vi "ep_Update Config Info (Waveform).vi"(6 "data length":i32, 7 "timing info":cluster{"t0":timestamp, "fs":sgl}, 8 "error in":errorcluster, 11 "task in":T1={"file refnums"=[], "Data Object"=refnum, "config info"={"station_name"="", "rec_dev_id"="", "rev_year"=1999.0, "TT"=0, "##A"=0, "##D"=0, "analog channel info"=[], "status channel info"=[], "lf"=-inf, "nrates"=65535, "samp info"=[], "initial timestamp"=timestamp(0 s since 1904-01-01), "trigger timestamp"=timestamp(0 s since 1904-01-01), "ft"=enum."Binary", "timemult"=1.0}, "public inf content"={"Source"="", "Record Type"=enum."Fault", "Phase ID"="", "Event Description"="", "Device ID"="", "Distance of Fault"=-1.0, "Distance Unit"=enum."Miles", "Max_Current"=inf, "Min_Current"=-inf, "Max_Voltage"=inf, "Min_Voltage"=-inf, "EventNoteCount"=0, "Event Information"=[]}, "private inf content"=[], "internal buffers"={"start index"=1, "config to public inf"=enum."disabled", "static config info"="", "static file_des record inf"="", "static file_des channel inf"="", "public inf"="", "private inf"=""}} {"public inf content"."Event Information"."min sample number" max=9999999999; "public inf content"."Event Information"."max sample number" max=9999999999; "config info"."nrates" max=999; "config info"."status channel info"."Dn" min=1 max=999999; "config info"."analog channel info"."An" min=1 max=999999; "config info"."trigger timestamp" format="%<%H:%M:%S%6u\n%d/%m/%Y>T"; "config info"."initial timestamp" format="%<%H:%M:%S%6u\n%d/%m/%Y>T"; "config info"."##D" max=999999; "config info"."##A" max=999999; "config info"."TT" min=1 max=999999; "config info"."rev_year" min=1999.0 max=1999.0}) -> (0 "error out":errorcluster, 3 "task out":T1={"file refnums"=[], "Data Object"=refnum, "config info"={"station_name"="", "rec_dev_id"="", "rev_year"=1999.0, "TT"=0, "##A"=0, "##D"=0, "analog channel info"=[], "status channel info"=[], "lf"=-inf, "nrates"=65535, "samp info"=[], "initial timestamp"=timestamp(0 s since 1904-01-01), "trigger timestamp"=timestamp(0 s since 1904-01-01), "ft"=enum."Binary", "timemult"=1.0}, "public inf content"={"Source"="", "Record Type"=enum."Fault", "Phase ID"="", "Event Description"="", "Device ID"="", "Distance of Fault"=-1.0, "Distance Unit"=enum."Miles", "Max_Current"=inf, "Min_Current"=-inf, "Max_Voltage"=inf, "Min_Voltage"=-inf, "EventNoteCount"=0, "Event Information"=[]}, "private inf content"=[], "internal buffers"={"start index"=1, "config to public inf"=enum."disabled", "static config info"="", "static file_des record inf"="", "static file_des channel inf"="", "public inf"="", "private inf"=""}} {"public inf content"."Event Information"."min sample number" max=9999999999; "public inf content"."Event Information"."max sample number" max=9999999999; "config info"."nrates" max=999; "config info"."status channel info"."Dn" min=1 max=999999; "config info"."analog channel info"."An" min=1 max=999999; "config info"."trigger timestamp" format="%<%H:%M:%S%6u\n%d/%m/%Y>T"; "config info"."initial timestamp" format="%<%H:%M:%S%6u\n%d/%m/%Y>T"; "config info"."##D" max=999999; "config info"."##A" max=999999; "config info"."TT" min=1 max=999999; "config info"."rev_year" min=1999.0 max=1999.0})   [LabVIEW 2011, in "NI_EP_COMTRADE.lvlib"]
uses:
  <vilib>/addons/Electrical Power/File IO/NI_EP_COMTRADE.lvlib
  <vilib>/addons/Electrical Power/File IO/COMTRADE/typedefs/ep_Task.ctl
  <vilib>/addons/Electrical Power/File IO/COMTRADE/typedefs/ep_Config Info.ctl
  <vilib>/addons/Electrical Power/File IO/COMTRADE/typedefs/ep_Analog Channel Info.ctl
  <vilib>/addons/Electrical Power/File IO/COMTRADE/typedefs/ep_Status Channel Info.ctl
  <vilib>/addons/Electrical Power/File IO/COMTRADE/typedefs/ep_File Format.ctl
  <vilib>/addons/Electrical Power/File IO/COMTRADE/typedefs/ep_Public Inf Content.ctl
  <vilib>/addons/Electrical Power/File IO/COMTRADE/typedefs/ep_Public Event Inf.ctl
  <vilib>/addons/Electrical Power/File IO/COMTRADE/typedefs/ep_Private Inf Content.ctl
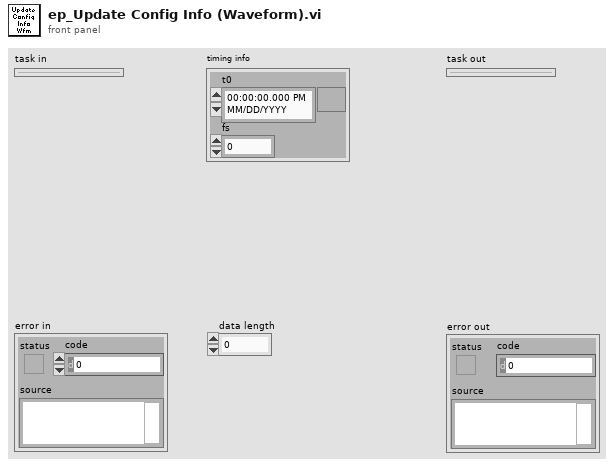
[diagram p1: front panel]
types:
  T1 = typedef "NI_EP_COMTRADE.lvlib/ep_Task.ctl" = cluster{"file refnums":refnum<file>[], "Data Object":refnum<k20>, "config info":T2, "public inf content":T6, "private inf content":T8, "internal buffers":cluster{"start index":u32, "config to public inf":enum16{"disabled", "enabled", "buffered"}, "static config info":string, "static file_des record inf":string, "static file_des channel inf":string, "public inf":string, "private inf":string}}
  T2 = typedef "NI_EP_COMTRADE.lvlib/ep_Config Info.ctl" = cluster{"station_name":string, "rec_dev_id":string, "rev_year":dbl, "TT":u32, "##A":u32, "##D":u32, "analog channel info":T3[], "status channel info":T4[], "lf":sgl, "nrates":u16, "samp info":cluster{"samp":sgl, "endsamp":u32}[], "initial timestamp":timestamp, "trigger timestamp":timestamp, "ft":T5, "timemult":sgl}
  T3 = typedef "NI_EP_COMTRADE.lvlib/ep_Analog Channel Info.ctl" = cluster{"An":u32, "ch_id":string, "ph":string, "ccbm":string, "uu":string, "a":sgl, "b":sgl, "skew":sgl, "min":i32, "max":i32, "primary":sgl, "secondary":sgl, "PS":enum16{"P", "S"}}
  T4 = typedef "NI_EP_COMTRADE.lvlib/ep_Status Channel Info.ctl" = cluster{"Dn":u32, "ch_id":string, "ph":string, "ccbm":string, "Y":bool}
  T5 = typedef "NI_EP_COMTRADE.lvlib/ep_File Format.ctl" = enum16{"ASCII", "Binary"}
  T6 = typedef "NI_EP_COMTRADE.lvlib/ep_Public Inf Content.ctl" = cluster{"Source":string, "Record Type":enum16{"Fault", "Unknown", "Misoperation", "Close", "Trip", "Reclose", "Power swing", "Simulation"}, "Phase ID":string, "Event Description":string, "Device ID":string, "Distance of Fault":dbl, "Distance Unit":enum16{"Miles", "Kilometers", "Percent of line", "Percent of setting", "Ohms"}, "Max_Current":dbl, "Min_Current":dbl, "Max_Voltage":dbl, "Min_Voltage":dbl, "EventNoteCount":u32, "Event Information":T7[]}
  T7 = typedef "NI_EP_COMTRADE.lvlib/ep_Public Event Inf.ctl" = cluster{"channel number":u32, "max value":dbl, "min value":dbl, "max sample number":u64, "min sample number":u64, "max sample text":string[], "min sample text":string[]}
  T8 = typedef "NI_EP_COMTRADE.lvlib/ep_Private Inf Content.ctl" = cluster{"Section Header":string, "Entry Names":string[], "Entry Values":string[]}[]
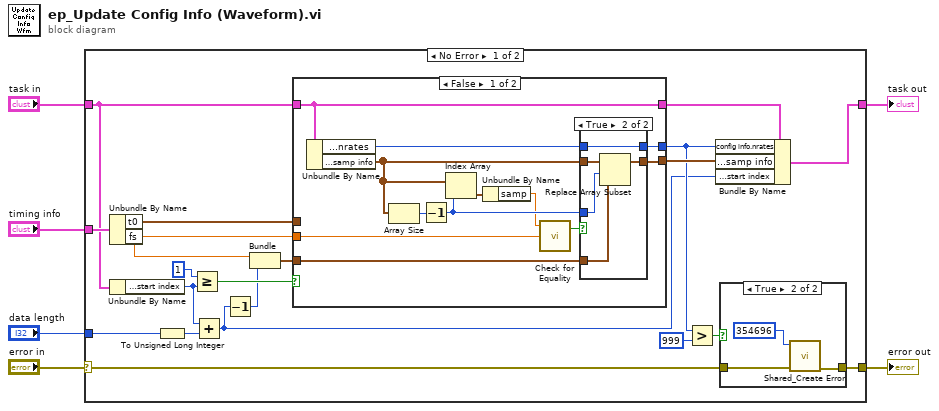
[diagram p0: block diagram]
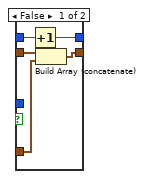
[diagram p3: hidden frame]
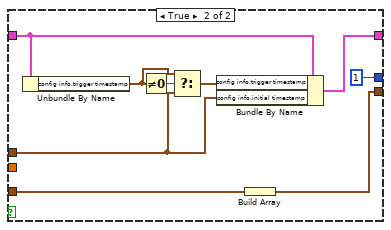
[diagram p4: hidden frame]
diagram:
  n1 = case shown="No Error" "error in" {
    selector: "error in" -> [w17 w62]
    tunnel: [w22 w63] -> w5
    tunnel: "task in" -> [w12 w63]
    tunnel: [w16 w62] -> w4
    tunnel: "data length" -> [w21 _]
    tunnel: "timing info" -> [w25 _]
    frame No Error {
      n2 = Unbundle By Name(w25) -> ("t0"=w23:timestamp, "fs"=w9:sgl)
      n3 = Unbundle By Name(w12) -> ("internal buffers.start index"=w7:u32)
      n4 = To Unsigned Long Integer(number=w21) -> (unsigned 32bit integer=w13:u32)
      n5 = Greater Or Equal?(x=u32 1, y=w7) -> (x >= y?=w14:bool)
      n6 = Add(x=w7, y=w13) -> (x+y=w10:u32)
      n7 = Decrement(x=w10) -> (x-1=w11:u32)
      n8 = Bundle("fs"=w9, w11) -> (w8:cluster{"fs":sgl, u32})  [unwired: 1 in]
      n9 = case shown="False" w14 {
        tunnel: [w38 w61] -> w26
        tunnel: w12 -> [w38 w58]
        tunnel: w23 -> [_ w54]
        tunnel: w9 -> [w34 _]
        tunnel: [w42 w60] -> w24
        tunnel: [w41 u16 1 ("nrates")] -> w20
        tunnel: w8 -> [w31 w53]
        frame False {
          n10 = Unbundle By Name(w38) -> ("config info.nrates"=w36:u16, "config info.samp info"=w37:cluster{"samp":sgl, "endsamp":u32}[])
          n11 = Array Size(array=w37) -> (size(s)=w40:i32)
          n12 = Decrement(x=w40) -> (x-1=w39:i32)
          n13 = Index Array(array=w37, index=w39) -> (element=w32:cluster{"samp":sgl, "endsamp":u32})
          n14 = Unbundle By Name(w32) -> ("samp"=w35:sgl)
          n15 = call <vilib>:"Check for Equality.vi"("n2"=w34, "n1"=w35) -> ("equal?"=w33:bool)  [unwired: 1 in, 1 out]
          n16 = case shown="True" w33 {
            tunnel: w37 -> [w47 w51]
            tunnel: [w46 w50] -> w42
            tunnel: [w45 w52] -> w41
            tunnel: w36 -> [w44 w52]
            tunnel: w39 -> [_ w49]
            tunnel: w31 -> [w43 w48]
            frame False {
              n17 = Increment(x=w44) -> (x+1=w45:u16)
              n18 = Build Array (concatenate)(w47, w43) -> (w46:cluster{"fs":sgl, "endsamp":u32}[])
            }
            frame True {
              n19 = Replace Array Subset(array=w51, new element=w48, index=w49) -> (w50:cluster{"samp":sgl, "endsamp":u32}[])
            }
          }
        }
        frame True {
          n20 = Unbundle By Name(w58) -> ("config info.trigger timestamp"=w55:timestamp)
          n21 = Not Equal To 0?(x=w55) -> (x != 0?=w57:bool)
          n22 = Select(t=w55, s=w57, f=w54) -> (s? t:f=w56:timestamp)
          n23 = Bundle By Name(cluster=w58, "config info.trigger timestamp"=w56, "config info.initial timestamp"=w54) -> (w61:T1)
          n24 = Build Array(w53) -> (w60:cluster{"fs":sgl, u32}[])
        }
      }
      n25 = Greater?(x=w20, y=u16 999) -> (0:w18:bool)
      n26 = Bundle By Name(cluster=w26, "config info.nrates"=w20, "config info.samp info"=w24, "internal buffers.start index"=w10) -> (w22:T1)
      n27 = case shown="True" w18 {
        tunnel: w17 -> [w27 w30]
        tunnel: [w27 w29] -> w16
        frame False {
        }
        frame True {
          n28 = call <vilib>:"Shared_Create Error.vi"("error in (no error)"=w30, "error code (0)"=354696 ("code")) -> ("error out"=w29:errorcluster)  [unwired: 9 in]
        }
      }
    }
    frame Error {
    }
  }
  "error out" <- w4
  "task out" <- w5
